vi "CRYGet Disable Device State.vi"(5 "O_Channel Info":T3[](array[typedef]) {"Coupling" items=["Default"=-1, "RSE"=10083, "NRSE"=10078, "Differential"=10106, "Pseudodifferential"=12529]; "term config" items=["Default"=-1, "RSE"=10083, "NRSE"=10078, "Differential"=10106, "Pseudodifferential"=12529]; "Anti-aliasing Factor (%fs)" format="%.2f"}, 7 "I_Channel Info":T3[](array[typedef]) {"Coupling" items=["Default"=-1, "RSE"=10083, "NRSE"=10078, "Differential"=10106, "Pseudodifferential"=12529]; "term config" items=["Default"=-1, "RSE"=10083, "NRSE"=10078, "Differential"=10106, "Pseudodifferential"=12529]; "Anti-aliasing Factor (%fs)" format="%.2f"}, 8 "O_Device Info In":T2(array[cluster]), 9 "I_Device Info In":T2(array[cluster]), 10 "Audio Driver":u32, 11 "In/Out":bool) -> (0 "All I/O_Device Info Out":T2(array[cluster]), 2 "Device Names":string[](array[string]), 3 "Disabled Items":i32[](array[numeric]))   [LabVIEW 2013]
uses:
  Typedef Control/CRYHardware Channel Info.ctl
panel:
  in  "Device Infor":T1
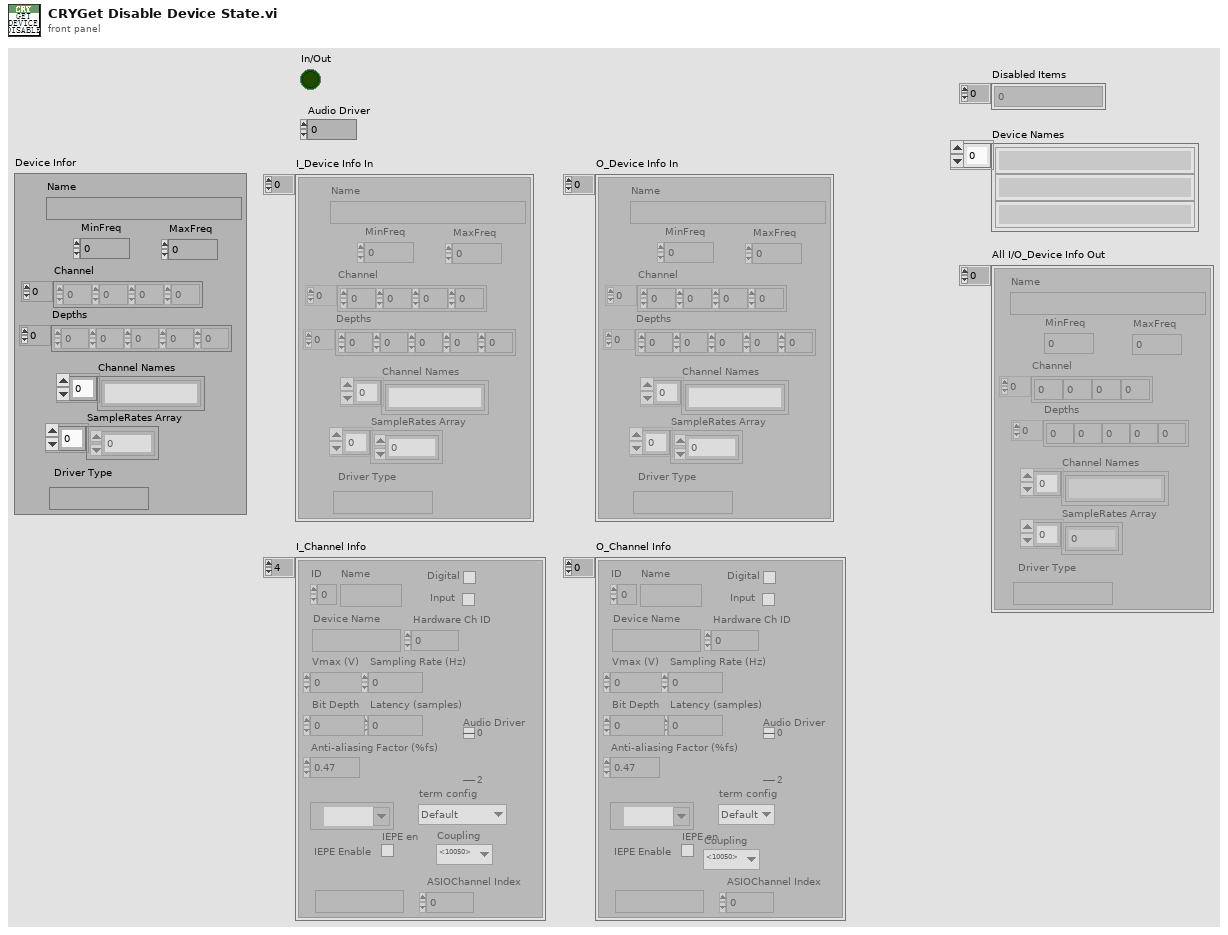
[diagram p1: front panel]
types:
  T1 = cluster{"Name":string, "MinFreq":dbl, "MaxFreq":dbl, "Channel":i32[], "Depths":i32[], "Channel Names":string[], "SampleRates Array":dbl[], "Driver Type":string}
  T2 = cluster{"Name":string, "MinFreq":dbl, "MaxFreq":dbl, "Channel":i32[], "Depths":i32[], "Channel Names":string[], "SampleRates Array":dbl[], "Driver Type":string}[]
  T3 = typedef "CRYHardware Channel Info.ctl" = cluster{"ID":i32, "Name":string, "Digital":bool, "Input":bool, "Device Name":string, "Hardware Ch ID":u8, "Vmax (V)":dbl, "Latency (samples)":dbl, "Sampling Rate (Hz)":u32, "Bit Depth":u32, "Anti-aliasing Factor (%fs)":sgl, "DAQmx Channel":tag, "term config":i32, "Coupling":i32, "IEPE en":bool, "ASIOChannel Name":string, "Audio Driver":u16, "ASIOChannel Index":u8}
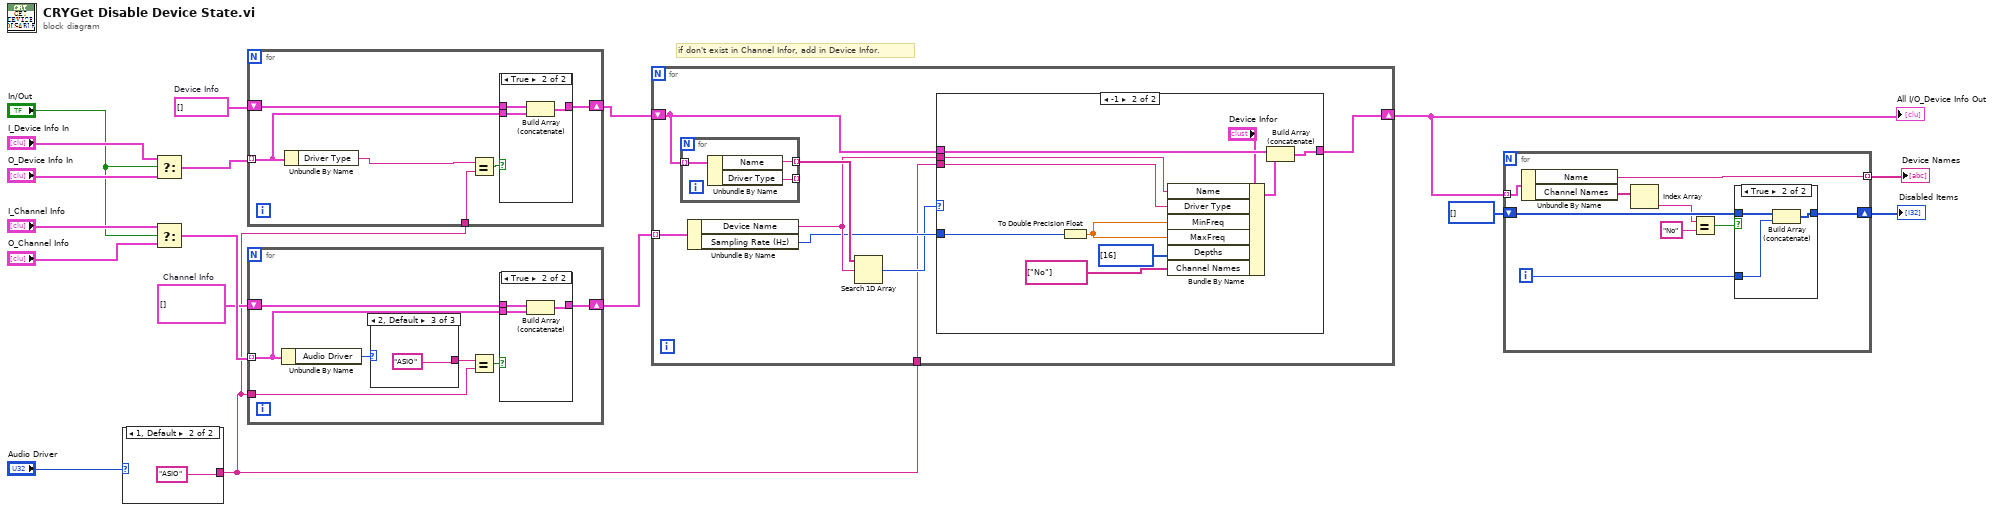
[diagram p0: block diagram]
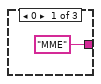
[diagram p4: hidden frame]
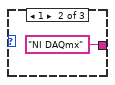
[diagram p5: hidden frame]
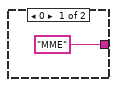
[diagram p7: hidden frame]
diagram:
  w3 = T2 []  # Device Info
  w7 = T3[] []  # Channel Info
  # "if don't exist in Channel Infor, add in Device Infor."
  n1 = case shown="1, Default" "Audio Driver" {
    tunnel: ["MME" ("Device Name") "ASIO" ("Device Name")] -> w2
    frame 0 {
    }
    frame 1, Default {
    }
  }
  n2 = Select(t="I_Device Info In", s="In/Out", f="O_Device Info In") -> (s? t:f=w4:T2)
  n3 = Select(t="I_Channel Info", s="In/Out", f="O_Channel Info") -> (s? t:f=w8:T3[])
  n4 = for {
    tunnel: w4 -> [w21] mode=indexing
    tunnel: w2 -> [w25]
    shift-right: [w22] -> w5
    shift-left: w3 -> [w23]
    n5 = Unbundle By Name(w21) -> ("Driver Type"=w20:string)
    n6 = Equal?(x=w20, y=w25) -> (x = y?=w24:bool)
    n7 = case shown="True" w24 {
      tunnel: w23 -> [w26 w29]
      tunnel: [w26 w28] -> w22
      tunnel: w21 -> [_ w27]
      frame False {
      }
      frame True {
        n8 = Build Array (concatenate)(w29, w27) -> (w28:T2)
      }
    }
  }
  n9 = for {
    tunnel: w8 -> [w30] mode=indexing
    tunnel: w2 -> [w34]
    shift-right: [w31] -> w6
    shift-left: w7 -> [w32]
    n10 = Unbundle By Name(w30) -> ("Audio Driver"=w36:u16)
    n11 = case shown="2, Default" w36 {
      tunnel: ["MME" ("Device Name") "NI DAQmx" ("Device Name") "ASIO" ("Device Name")] -> w35
      frame 0 {
      }
      frame 1 {
      }
      frame 2, Default {
      }
    }
    n12 = Equal?(x=w35, y=w34) -> (x = y?=w33:bool)
    n13 = case shown="True" w33 {
      tunnel: w32 -> [w37 w40]
      tunnel: [w37 w39] -> w31
      tunnel: w30 -> [_ w38]
      frame False {
      }
      frame True {
        n14 = Build Array (concatenate)(w40, w38) -> (w39:T3[])
      }
    }
  }
  n15 = for {
    tunnel: w6 -> [w51] mode=indexing
    shift-right: [w50] -> w10
    shift-left: w5 -> [w49]
    tunnel: w2 -> [w44]
    n16 = for {
      tunnel: w49 -> [w65] mode=indexing
      tunnel: [w64] -> w48 mode=indexing
      tunnel: [w63] -> _ mode=indexing
      n17 = Unbundle By Name(w65) -> ("Name"=w64:string, "Driver Type"=w63:string)
    }
    n18 = Unbundle By Name(w51) -> ("Device Name"=w47:string, "Sampling Rate (Hz)"=w46:u32)
    n19 = Search 1D Array(1D array=w48, element=w47) -> (index of element=w45:i32)  [unwired: 1 in]
    n20 = case shown="-1" w45 {
      tunnel: w49 -> [w52 w62]
      tunnel: [w52 w61] -> w50
      tunnel: w47 -> [_ w59]
      tunnel: w44 -> [_ w57]
      tunnel: w46 -> [_ w56]
      frame 0, Default {
      }
      frame -1 {
        n21 = To Double Precision Float(number=w56) -> (double precision float=w55:dbl)
        n22 = Bundle By Name(cluster="Device Infor", "Name"=w59, "Driver Type"=w57, "MinFreq"=w55, "MaxFreq"=w55, "Depths"=i32[] [16], "Channel Names"=string[] ["No"]) -> (w58:T1)
        n23 = Build Array (concatenate)(w62, w58) -> (w61:T2)
      }
    }
  }
  "All I/O_Device Info Out" <- w10
  n24 = for {
    shift-right: [w72] -> w16
    shift-left: i32[] [] ("Disabled Items") -> [w73]
    tunnel: w10 -> [w71] mode=indexing
    tunnel: [w66] -> w1 mode=indexing
    i -> [w74]
    n25 = Unbundle By Name(w71) -> ("Name"=w66:string, "Channel Names"=w70:string[])
    n26 = Index Array(array=w70) -> (element=w69:string)  [unwired: 1 in]
    n27 = Equal?(x=w69, y="No" ("return type")) -> (x = y?=w67:bool)
    n28 = case shown="True" w67 {
      tunnel: w74 -> [_ w77]
      tunnel: w73 -> [w75 w78]
      tunnel: [w75 w76] -> w72
      frame False {
      }
      frame True {
        n29 = Build Array (concatenate)(w78, w77) -> (w76:i32[])
      }
    }
  }
  "Disabled Items" <- w16
  "Device Names" <- w1
